vi "HEWH Runtime Wh Reset.vi"(7 "Power Analyzer":T1, 8 "error in (no error)":errorcluster, 9 "Yokogawa WT210":refnum<visa-resource-name>, 10 "MW100":refnum<visa-resource-name>, 11 "Reset Timer":bool) -> (0 "error out":errorcluster)   [LabVIEW 2016]
uses:
  Utility/Type Definitions/UTILITY Power Analyzer.ctl
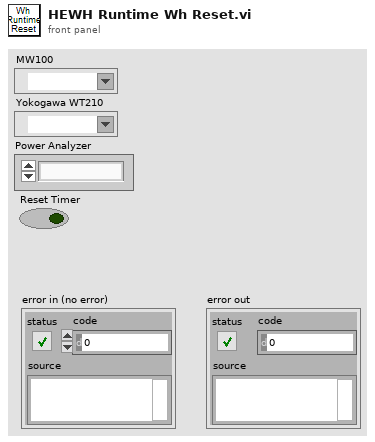
[diagram p1: front panel]
types:
  T1 = typedef "UTILITY Power Analyzer.ctl" = enum16{"", "APLUS", "WT210", "WT500", "WT300", "OSI", "Debug", "WT230", "WT300_1", "WT300_2"}
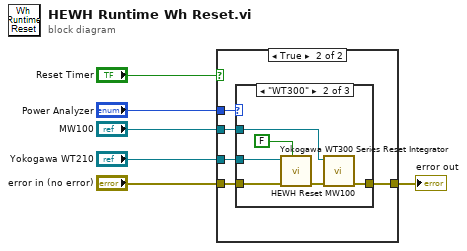
[diagram p0: block diagram]
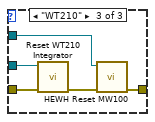
[diagram p4: hidden frame]
diagram:
  n1 = case shown="True" "Reset Timer" {
    tunnel: "Power Analyzer" -> [_ w12]
    tunnel: "error in (no error)" -> [w7 w11]
    tunnel: [w7 w10] -> w5
    tunnel: "Yokogawa WT210" -> [_ w9]
    tunnel: "MW100" -> [_ w8]
    frame False {
    }
    frame True {
      n2 = case shown="\"WT300\"" w12 {
        tunnel: w11 -> [w13 w18 w24]
        tunnel: [w13 w15 w21] -> w10
        tunnel: w9 -> [_ w17 w23]
        tunnel: w8 -> [_ w14 w20]
        frame "", Default {
        }
        frame "WT300" {
          n3 = call "Yokogawa WT300 Series Reset Integrator.vi"("Initialization Routing?"=FALSE, "Error In"=w18, "VISA Refnum in"=w17) -> ("Error Out"=w16:errorcluster)  [unwired: 7 in, 1 out]
          n4 = call "HEWH Reset MW100.vi"("error in (no error)"=w16, "MW100 VISA In"=w14) -> ("error out"=w15:errorcluster)  [unwired: 8 in, 1 out]
        }
        frame "WT210" {
          n5 = call "Reset WT210 Integrator.vi"("error in (no error)"=w24, "VISA resource name"=w23) -> ("error out"=w22:errorcluster)  [unwired: 8 in, 1 out]
          n6 = call "HEWH Reset MW100.vi"("error in (no error)"=w22, "MW100 VISA In"=w20) -> ("error out"=w21:errorcluster)  [unwired: 8 in, 1 out]
        }
      }
    }
  }
  "error out" <- w5
